vi "On Load Action VI.vi"(8 "error in (no error)":errorcluster, 11 "Device Item Ref in":T1 format="%.0x") -> (0 "error out":errorcluster, 3 "Device Item Ref out":T1 format="%.0x")   [LabVIEW 2023, in "NI 272x Resistive Simulation Custom Device Configuration.lvlib"]
uses:
  NI 272x Resistive Simulation Custom Device Configuration.lvlib
  <vilib>/NI VeriStand/Custom Device API/Custom Device Item Ref.ctl
  <vilib>/NI VeriStand/Custom Device API/Custom Device API.lvlib
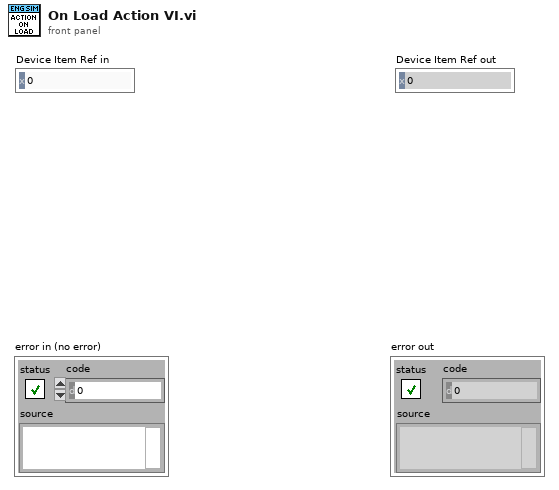
[diagram p1: front panel]
types:
  T1 = typedef "Custom Device API.lvlib/Custom Device Item Ref.ctl" = u64
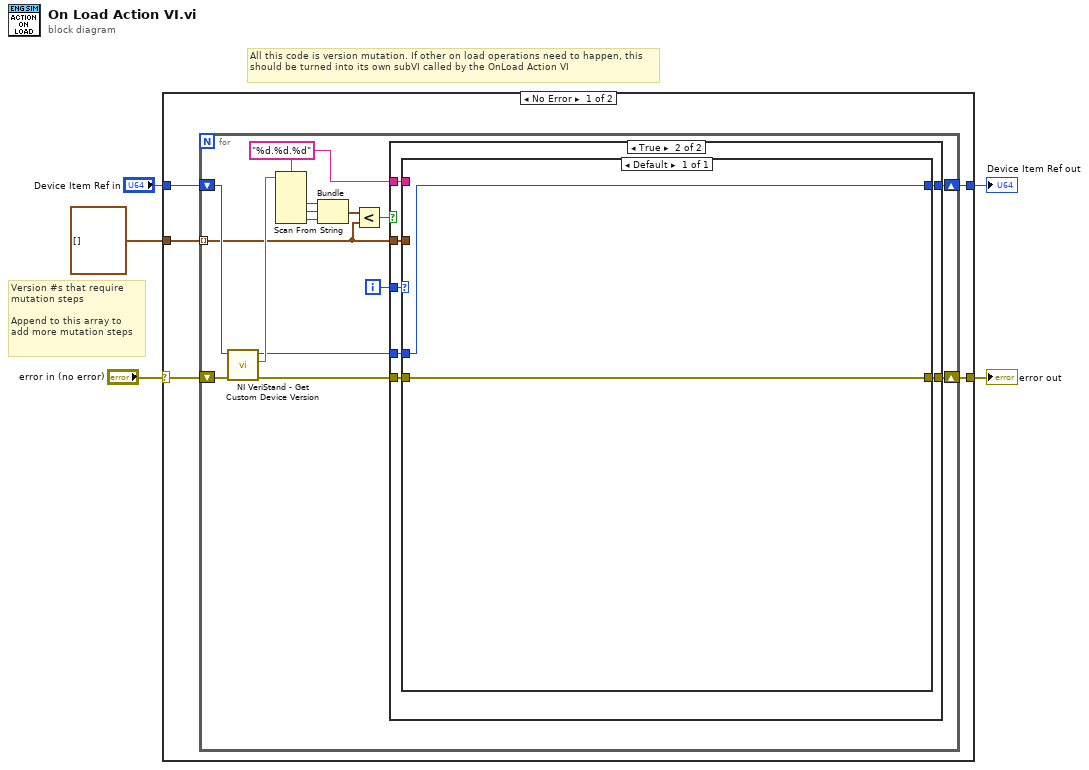
[diagram p0: block diagram]
diagram:
  # "All this code is version mutation. If other on load operations need to happen, this should be turned into its own subVI called by the OnLoad Action VI"
  # "Version #s that require\nmutation steps\n\nAppend to this array to\nadd more mutation steps"
  n1 = case shown="No Error" "error in (no error)" {
    selector: "error in (no error)" -> [w9 w38]
    tunnel: [w6 w38] -> w4
    tunnel: "Device Item Ref in" -> [w8 w37]
    tunnel: [w7 w37] -> w2
    tunnel: cluster{i32, i32, i32}[] [] -> [w10 _]
    frame No Error {
      n2 = for {
        tunnel: w10 -> [w13] mode=indexing
        shift-right: [w18] -> w6
        shift-left: w9 -> [w23]
        shift-right: [w16] -> w7
        shift-left: w8 -> [w22]
        i -> [w15]
        w14 = "%d.%d.%d" ("format string")
        n3 = call <vilib>:"NI VeriStand - Get Custom Device Version.vi"("error in (no error)"=w23, "Device Ref in"=w22) -> ("error out"=w19:errorcluster, "Value"=w21:string, "Device Ref out"=w17:T1)  [unwired: 7 in]
        n4 = Scan From String(format string=w14, input string=w21) -> (output 1=w24:i32, output 2=w25:i32, output 3=w12:i32)  [unwired: 5 in, 3 out]
        n5 = Bundle(w24, w25, w12) -> (w11:cluster{i32, i32, i32})  [unwired: 1 in]
        n6 = Less?(x=w11, y=w13) -> (x < y?=w20:bool)
        n7 = case shown="True" w20 {
          tunnel: w19 -> [w27 w34]
          tunnel: [w27 w33] -> w18
          tunnel: w17 -> [w26 w30]
          tunnel: [w26 w31] -> w16
          tunnel: w15 -> [_ w32]
          tunnel: w13 -> [_ w29]
          tunnel: w14 -> [_ w28]
          frame False {
          }
          frame True {
            n8 = case shown="Default" w32 {
              tunnel: w34 -> [w36]
              tunnel: [w36] -> w33
              tunnel: [w35] -> w31
              tunnel: w30 -> [w35]
              tunnel: w29 -> [_]
              tunnel: w28 -> [_]
              frame Default {
              }
            }
          }
        }
      }
    }
    frame Error {
    }
  }
  "error out" <- w4
  "Device Item Ref out" <- w2
